vi "Close Hardware.vi"(8 "error in (no error)":errorcluster, 11 "Instrument.SR7270 in":refnum<class "Instrument.SR7270.lvclass">) -> (0 "error out":errorcluster, 3 "Instrument.SR7270 out":refnum<class "Instrument.SR7270.lvclass">)   [LabVIEW 2019, in "Instrument.SR7270.lvclass"]
uses:
  Instrument.SR7270.lvclass
  Instrument.SR7270.lvclass/Instrument.SR7270.ctl
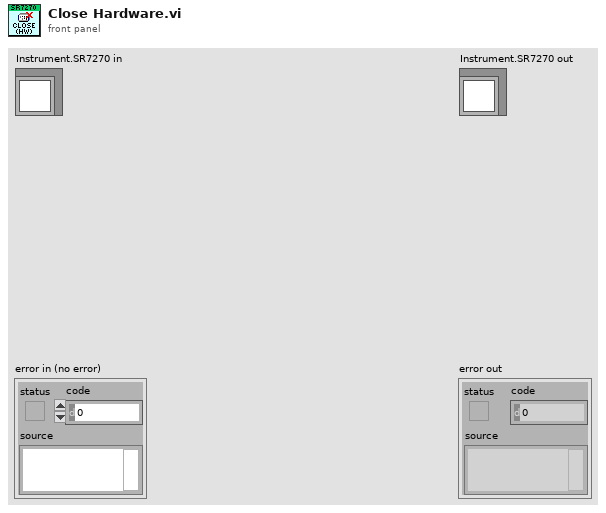
[diagram p1: front panel]
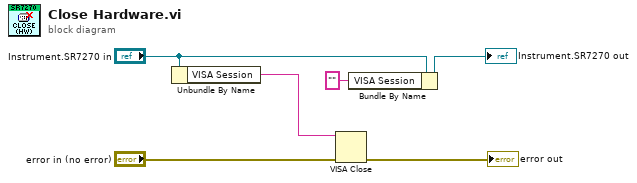
[diagram p0: block diagram]
diagram:
  n1 = Unbundle By Name("Instrument.SR7270 in") -> ("VISA Session"=w6:string)
  n2 = VISA Close(VISA resource name=w6, error in (no error)="error in (no error)") -> (error out=→"error out":errorcluster)
  n3 = Bundle By Name(cluster="Instrument.SR7270 in", "VISA Session"="") -> (→"Instrument.SR7270 out":refnum<class "Instrument.SR7270.lvclass">)
